vi "General Linear Fit.vi"(0 "Y":dbl[](array[numeric]), 1 "covariance selector":T4(ring), 5 "H":dbl[][](array[numeric]), 7 "Weight":dbl[](array[numeric]), 9 "tolerance":dbl=0.0001, 11 "method":T1 items=["Least Square", "Least Absolute Residual", "Bisquare"], 13 "algorithm":T3 items=["SVD", "Givens", "Givens2", "Householder", "LU Decomposition", "Cholesky", "SVD for Rank Deficient H"]) -> (4 "Best Fit":dbl[](array[numeric]), 6 "Coefficients":dbl[](array[numeric]), 8 "Covariance":T2, 14 "residue":dbl, 15 "error":i32)   [LabVIEW 2010, in "NI_AALPro.lvlib"]
doc: "Finds the k-dimension linear curve values and the set of k-dimension linear fit coefficients, which describe the k-dimension linear curve that best represents the input data set using the Least Square, Least Absolute Residual, or Bisquare method."
uses:
  NI_AALPro.lvlib
  General Linear Fit Algorithm.ctl
  RealMatrix.ctl
  Curve Fitting Criteria.ctl
  NI_Matrix.lvlib
panel:
  # "General Linear Fit"
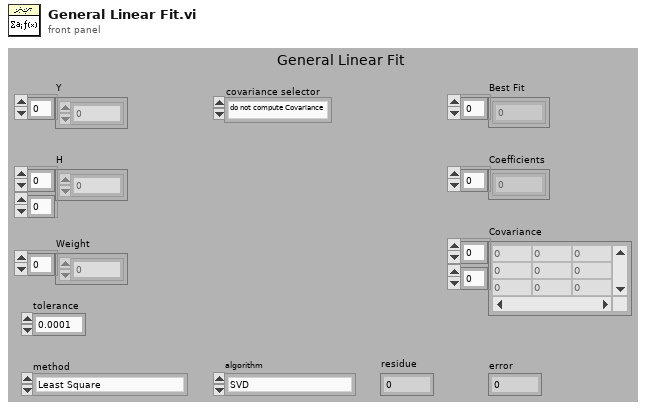
[diagram p1: front panel]
types:
  T1 = typedef "NI_AALPro.lvlib/Curve Fitting Criteria.ctl" = u16
  T2 = typedef "NI_Matrix.lvlib/RealMatrix.ctl" = dbl[][]
  T3 = typedef "NI_AALPro.lvlib/General Linear Fit Algorithm.ctl" = u16
  T4 = enum32{"do not compute Covariance", " compute Covariance"}
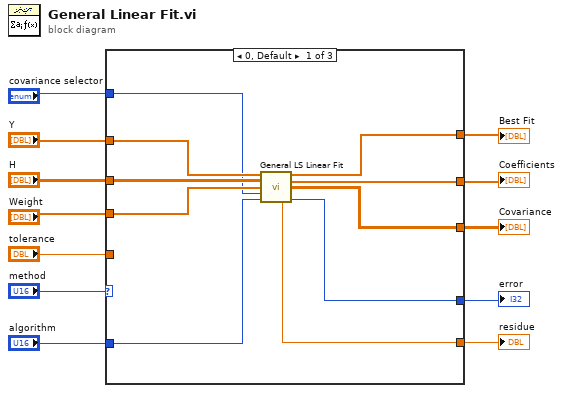
[diagram p0: block diagram]
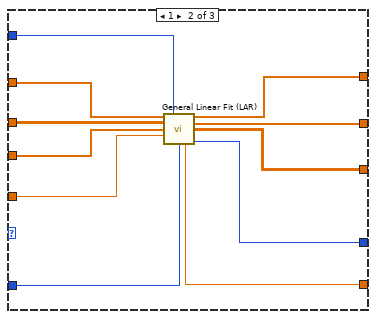
[diagram p2: hidden frame]
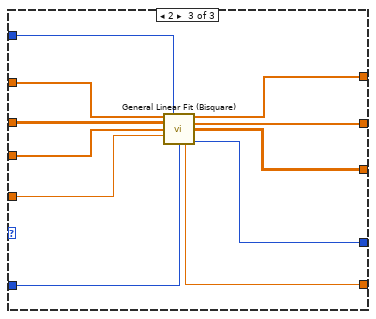
[diagram p3: hidden frame]
diagram:
  n1 = case shown="0, Default" "method" {
    tunnel: "H" -> [w22 w33 w44]
    tunnel: "Y" -> [w21 w32 w43]
    tunnel: "Weight" -> [w20 w31 w42]
    tunnel: "covariance selector" -> [w13 w23 w34]
    tunnel: "algorithm" -> [w14 w24 w35]
    tunnel: [w19 w30 w41] -> w6
    tunnel: [w18 w29 w40] -> w5
    tunnel: [w17 w28 w39] -> w4
    tunnel: [w16 w27 w38] -> w3
    tunnel: [w15 w26 w37] -> w2
    tunnel: "tolerance" -> [_ w25 w36]
    frame 0, Default {
      n2 = call "General LS Linear Fit.vi"("Y"=w21, "H"=w22, "Weight"=w20, "covariance selector"=w13, "algorithm"=w14) -> ("Best Fit"=w19:dbl[], "Coefficients"=w18:dbl[], "Covariance"=w17:T2, "mse"=w15:dbl, "error"=w16:i32)  [unwired: 6 out]
    }
    frame 1 {
      n3 = call "General Linear Fit (LAR).vi"("Y"=w32, "covariance selector"=w23, "H"=w33, "Weight"=w31, "tolerance"=w25, "algorithm"=w24) -> ("Best Fit"=w30:dbl[], "Coefficients"=w29:dbl[], "Covariance"=w28:T2, "residue"=w26:dbl, "error"=w27:i32)  [unwired: 1 in, 4 out]
    }
    frame 2 {
      n4 = call "General Linear Fit (Bisquare).vi"("Y"=w43, "covariance selector"=w34, "H"=w44, "Weight"=w42, "tolerance"=w36, "algorithm"=w35) -> ("Best Fit"=w41:dbl[], "Coefficients"=w40:dbl[], "Covariance"=w39:T2, "residue"=w37:dbl, "error"=w38:i32)  [unwired: 1 in, 4 out]
    }
  }
  "Best Fit" <- w6
  "Coefficients" <- w5
  "Covariance" <- w4
  "residue" <- w2
  "error" <- w3
